vi "MessageName.vi"() -> (2 "MessageName":string)   [LabVIEW 2020, in "TcpPayload.lvlib"]
uses:
  TcpPayload.lvlib
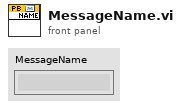
[diagram p1: front panel]
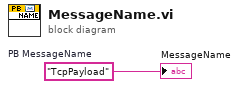
[diagram p0: block diagram]
diagram:
  w1 = "TcpPayload"  # PB MessageName
  "MessageName" <- w1
